vi "Status ConvBox Handler.vi"(8 "error in(no error)":errorcluster, 10 "Value In":string, 11 "Listener in":refnum<class "Listener.lvclass">) -> (0 "error out":errorcluster, 3 "Listener out":refnum<class "Listener.lvclass">)   [LabVIEW 2019, in "Listener.lvclass"]
uses:
  Listener.lvclass
  Listener.lvclass/Listener.ctl
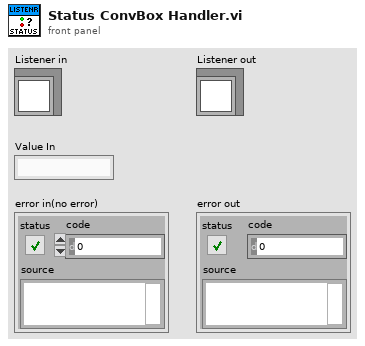
[diagram p1: front panel]
types:
  T1 = typedef "Listener.lvclass/RS-xxx To GPIB ConvBox Data Structure.ctl" = cluster{"Data":string, "Command Messages Read":string[], "Address":string, "Data Length":u32}
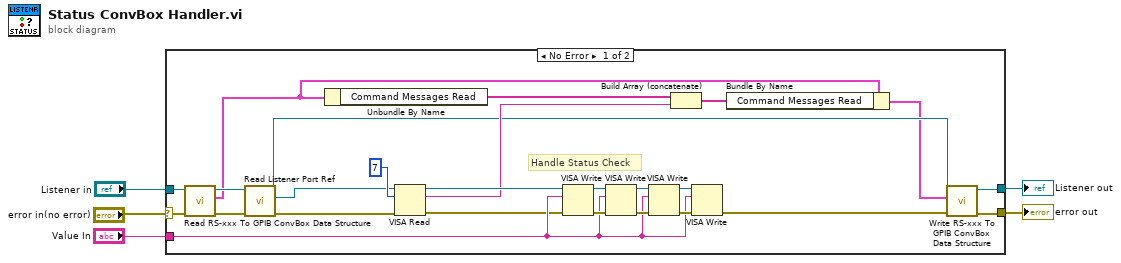
[diagram p0: block diagram]
diagram:
  n1 = case shown="No Error" "error in(no error)" {
    selector: "error in(no error)" -> [w17 w32]
    tunnel: "Value In" -> [w25 _]
    tunnel: [w6 w32] -> w4
    tunnel: "Listener in" -> [w18 w31]
    tunnel: [w7 w31] -> w1
    frame No Error {
      # "Handle Status Check"
      n2 = call-dynamic "Read RS-xxx To GPIB ConvBox Data Structure.vi"("error in (no error)"=w17, "Listener in"=w18) -> ("error out"=w15:errorcluster, "RS-xxx To GPIB ConvBox Data Structure"=w10:T1, "Listener out"=w16:refnum<class "Listener.lvclass">)  [unwired: 7 in]
      n3 = call "Read Listener Port Ref.vi"("error in (no error)"=w15, "Listener in"=w16) -> ("error out"=w20:errorcluster, "Listener Port Ref"=w19:refnum<visa-resource-name>, "Listener out"=w11:refnum<class "Listener.lvclass">)  [unwired: 7 in]
      n4 = Unbundle By Name(w10) -> ("Command Messages Read"=w14:string[])
      n5 = VISA Read(VISA resource name=w19, byte count=u32 7, error in (no error)=w20) -> (VISA resource name out=w22:refnum<visa-resource-name>, read buffer=w13:string, error out=w23:errorcluster)  [unwired: 1 out]
      n6 = VISA Write(VISA resource name=w22, write buffer=w25, error in (no error)=w23) -> (VISA resource name out=w29:refnum<visa-resource-name>, error out=w30:errorcluster)  [unwired: 1 out]
      n7 = VISA Write(VISA resource name=w29, write buffer=w25, error in (no error)=w30) -> (VISA resource name out=w27:refnum<visa-resource-name>, error out=w28:errorcluster)  [unwired: 1 out]
      n8 = VISA Write(VISA resource name=w27, write buffer=w25, error in (no error)=w28) -> (VISA resource name out=w24:refnum<visa-resource-name>, error out=w26:errorcluster)  [unwired: 1 out]
      n9 = Build Array (concatenate)(w14, w13) -> (w9:string[])
      n10 = VISA Write(VISA resource name=w24, write buffer=w25, error in (no error)=w26) -> (error out=w12:errorcluster)  [unwired: 2 out]
      n11 = Bundle By Name(cluster=w10, "Command Messages Read"=w9) -> (w8:T1)
      n12 = call-dynamic "Write RS-xxx To GPIB ConvBox Data Structure.vi"("error in (no error)"=w12, "RS-xxx To GPIB ConvBox Data Structure"=w8, "Listener in"=w11) -> ("error out"=w6:errorcluster, "Listener out"=w7:refnum<class "Listener.lvclass">)  [unwired: 7 in]
    }
    frame Error {
    }
  }
  "error out" <- w4
  "Listener out" <- w1
